vi "CAN发车速.vi"() -> ()   [LabVIEW 2020]
uses:
  Other/ZLG_CAN/Snap7/lib/Snap7.lvlib
  Other/ZLG_CAN/ZLG_CAN.lvlib
panel:
  in  "周期(ms)":u32=10 min=1 format="%d ms"
  in  "帧格式":enum16{"数据帧", "远程帧"}(ring)
  in  "帧类型":enum8{"标准帧", "扩展帧"}(ring)
  in  "ID":u32 format="0x%x"
  in  "波特率":u32(ring)=11 items=["5Kbps", "10Kbps", "20Kbps", "40Kbps", "50Kbps", "80Kbps", "100Kbps", "125Kbps", "200Kbps", "250Kbps", "400Kbps", "500Kbps", "666Kbps", "800Kbps", "1000Kbps"]
  in  "CAN 通道":u32(ring) items=["0", "1"]
  in  "索引":u32(ring) items=["0", "1", "2", "3", "4", "5", "6", "7", "8"]
  in  "设备类型":u32(ring)=3 items=["PCI5121"=1, "PCI9810"=2, "USBCAN1"=3, "USBCAN2"=4, "PCI9820"=5, "PCI5110"=7, "PC104CAN"=11, "CANETUDP"=12, "PCI9840B"=14, "PC104C2"=15, "PCI9820I"=16, "CANETTCP"=17, "PCIE9221"=24, "PCI5010U"=19, "USBCAN_E_U"=20, "USBCAN_2E_U"=21, "PCI5020U"=22, "PCIE9120I"=27, "PCIE9110I"=28, "PCIE9140I"=29]
  out "?":string
  out "Running":bool
  out "Status":string="No Error"
  in  "Word Length":i32(ring)=2 items=["Bit"=1, "Byte"=2, "Word"=4, "DWord"=6, "Real"=8, "Counter"=28, "Timer"=29]
  in  "Area":i32(ring)=132 items=["Inputs (EB)"=129, "Output (AB)"=130, "Bit Memory (M)"=131, "Data (DB)"=132, "Counters (Z)"=28, "Timers (T)"=29]
  in  "Amount":i32=1
  in  "Start":i32
  in  "DB Number":i32=1
  out "Data":u8[](array[numeric])
  in  "Stop":bool
  in  "Slot":i32=1
  in  "Rack":i32
  in  "Address IP":string="192.168.0.21"
  # "Data Read"
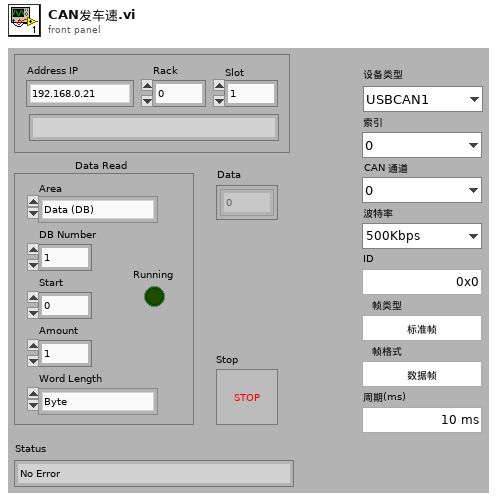
[diagram p1: front panel]
types:
  T1 = enum16{"big-endian, network order", "native, host order", "little-endian"}
  T2 = typedef "ZLG_CAN.lvlib/Start_CAN (Reply Payload)--cluster.ctl" = cluster{"Success":bool, "Start_CAN_error":errorcluster}
  T3 = cluster{u8, u8, "y":u8, "y":u8, "y":u8, "y":u8, "y":u8, "y":u8}
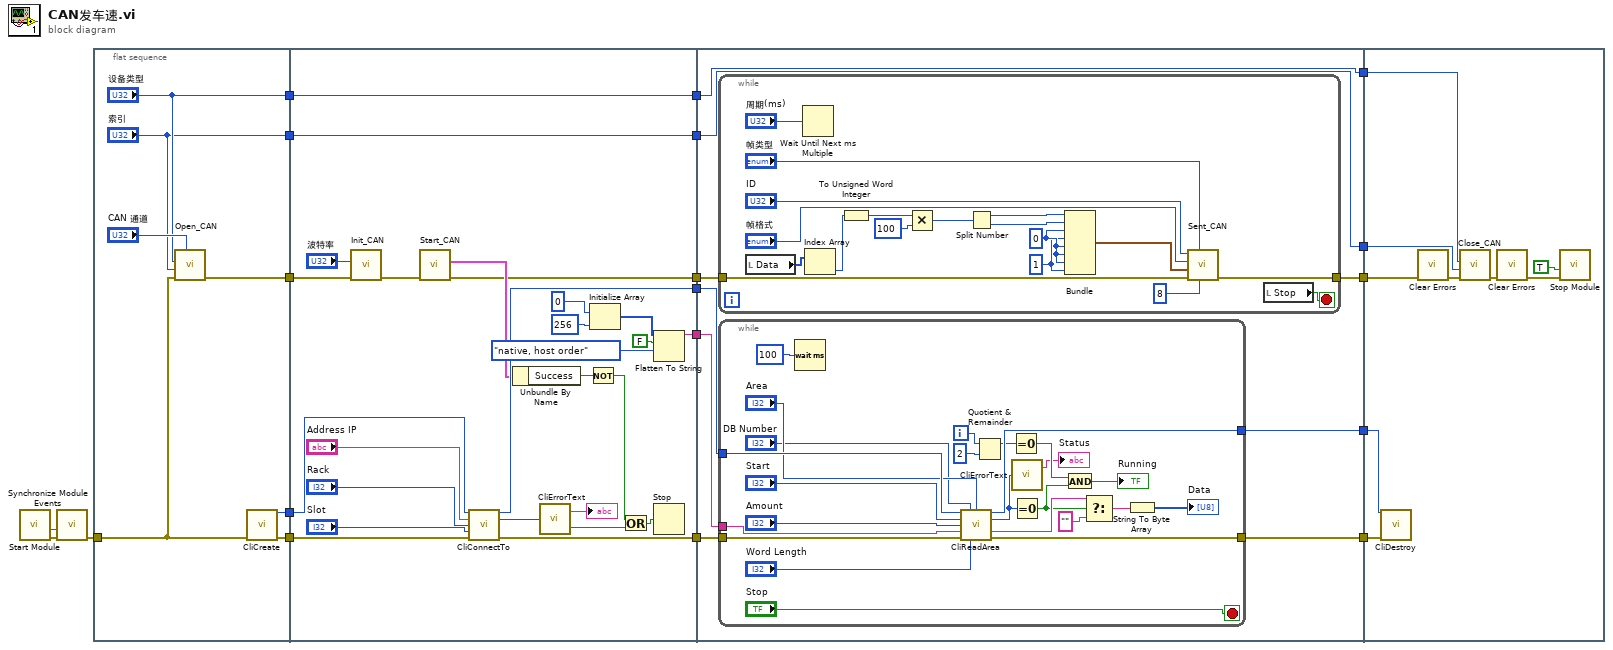
[diagram p0: block diagram]
diagram:
  n1 = call "Start Module.vi"() -> ("error out"=w12:errorcluster, "Wait for Event Sync?"=w11:bool)  [unwired: 8 in, 2 out]
  n2 = call "Synchronize Module Events.vi"("error in (no error)"=w12, "Wait for Event Sync?"=w11) -> ("error out"=w10:errorcluster)  [unwired: 9 in]
  n3 = flat-sequence {
    tunnel: [w26] -> w16
    tunnel: [w25] -> w15
    tunnel: w10 -> [w21]
    tunnel: ["索引"] -> w3
    tunnel: ["设备类型"] -> w2
    tunnel: [w22] -> w1
    tunnel: [w47] -> w19
    tunnel: [w40] -> w18
    tunnel: [w46] -> w17
    tunnel: w16 -> [w42]
    tunnel: w15 -> [w41]
    tunnel: [w36] -> w9
    tunnel: [w30] -> w7
    tunnel: [w31] -> w5
    tunnel: w3 -> [w31]
    tunnel: w2 -> [w30]
    tunnel: w1 -> [w29]
    tunnel: w19 -> [w61]
    tunnel: w18 -> [w60]
    tunnel: w17 -> [w59]
    tunnel: [w58] -> w14
    tunnel: [w57] -> w13
    tunnel: w9 -> [w56]
    tunnel: [w55] -> w8
    tunnel: w7 -> [w54]
    tunnel: [w54] -> w6
    tunnel: w5 -> [w53]
    tunnel: [w53] -> w4
    tunnel: w14 -> [w112]
    tunnel: w13 -> [w111]
    tunnel: w8 -> [w110]
    tunnel: w6 -> [w109]
    tunnel: w4 -> [w108]
    frame #0 {
      n4 = call "Open_CAN.vi"("CAN 通道"="CAN 通道", "error in (no error)"=w21, "索引"="索引", "设备类型"="设备类型") -> ("error out"=w22:errorcluster)  [unwired: 7 in]
      n5 = call "CliCreate.vi"("error in (no error)"=w21) -> ("ref out"=w26:u64, "error out"=w25:errorcluster)  [unwired: 13 in]
    }
    frame #1 {
      n6 = call "Init_CAN.vi"("error in (no error)"=w29, "波特率"="波特率") -> ("error out"=w32:errorcluster)  [unwired: 9 in]
      n7 = call "Start_CAN.vi"("error in (no error)"=w32) -> ("error out"=w36:errorcluster, "Reply Payload"=w37:T2)  [unwired: 8 in, 1 out]
      n8 = call "CliConnectTo.vi"("ref in"=w42, "Address"="Address IP", "Rack"="Rack", "Slot"="Slot", "error in (no error)"=w41) -> ("ref out"=w40:u64, "Result"=w38:i32, "error out"=w47:errorcluster)  [unwired: 8 in]
      n9 = Unbundle By Name(w37) -> ("Success"=w35:bool)
      n10 = call "CliErrorText.vi"("ErrNo"=w38) -> ("Error"=w34:bool, "ErrMessage"=→"?":string)
      n11 = Not(x=w35) -> (.not. x?=w27:bool)
      n12 = Initialize Array(u8 0, 256) -> (w50:u8[])
      n13 = Or(x=w27, y=w34) -> (x .or. y?=w33:bool)
      n14 = Flatten To String(anything=w50, prepend array or string size? (T)=FALSE, byte order (0:big-endian, network order)=T1."native, host order") -> (data string=w46:string)  [unwired: 1 in, 2 out]
      n15 = Stop(stop? (T)=w33) -> ()
    }
    frame #2 {
      n16 = while {
        tunnel: w56 -> [w79]
        tunnel: [w77] -> w55
        stop <- w78 stop-if-true
        w68 = u8 1 ("y")
        w69 = u8 0 ("y")
        n17 = local read "Data"() -> (w76:u8[])
        n18 = Wait Until Next ms Multiple(millisecond multiple="周期(ms)") -> ()  [unwired: 1 out]
        n19 = Index Array(array=w76) -> (element=w75:u8)  [unwired: 1 in]
        n20 = To Unsigned Word Integer(number=w75) -> (unsigned 16bit integer=w73:u16)
        n21 = Multiply(x=w73, y=u16 100) -> (x*y=w72:u16)
        n22 = Split Number(x=w72) -> (hi(x)=w71:u8, lo(x)=w70:u8)
        n23 = Bundle(w71, w70, "y"=w69, "y"=w68, "y"=w69, "y"=w69, "y"=w69, "y"=w68) -> (w67:T3)  [unwired: 1 in]
        n24 = call "Sent_CAN.vi"("帧长度"=u8 8, "帧类型"="帧类型", "error in (no error)"=w79, "帧数据"=w67, "帧格式"="帧格式", "ID"="ID") -> ("error out"=w77:errorcluster)  [unwired: 5 in]
        n25 = local read "Stop"() -> (w78:bool)
      }
      n26 = while {
        tunnel: w61 -> [w102]
        tunnel: w60 -> [w101]
        tunnel: w59 -> [w100]
        tunnel: [w94] -> w58
        tunnel: [w93] -> w57
        i -> [w91]
        stop <- "Stop" stop-if-true
        n27 = Wait (ms)(milliseconds to wait=u32 100 ("Loop Delay (ms)")) -> ()  [unwired: 1 out]
        n28 = call "CliReadArea.vi"("ref in"=w101, "DB Number"="DB Number", "Area"="Area", "Start"="Start", "Amount"="Amount", "data in"=w100, "error in (no error)"=w102, "Word Length"="Word Length") -> ("ref out"=w94:u64, "Result"=w92:i32, "data out"=w85:string, "error out"=w93:errorcluster)  [unwired: 4 in]
        n29 = Quotient & Remainder(x=w91, y=2) -> (x-y*floor(x/y)=w89:i32)  [unwired: 1 out]
        n30 = Equal To 0?(x=w89) -> (x = 0?=w88:bool)
        n31 = call "CliErrorText.vi"("ErrNo"=w92) -> ("ErrMessage"=→"Status":string)  [unwired: 1 out]
        n32 = Equal To 0?(x=w92) -> (x = 0?=w84:bool)
        n33 = And(x=w88, y=w84) -> (x .and. y?=→"Running":bool)
        n34 = Select(t=w85, s=w84, f="") -> (s? t:f=w82:string)
        n35 = String To Byte Array(string=w82) -> (unsigned byte array=→"Data":u8[])
      }
    }
    frame #3 {
      n36 = call "CliDestroy.vi"("ref in"=w112, "error in (no error)"=w111) -> ()  [unwired: 13 in, 1 out]
      n37 = call <vilib>:"Clear Errors.vi"("error in (no error)"=w110) -> ("error out"=w104:errorcluster)  [unwired: 5 in, 1 out]
      n38 = call "Close_CAN.vi"("error in (no error)"=w104, "索引"=w108, "设备类型"=w109) -> ("error out"=w107:errorcluster)  [unwired: 8 in]
      n39 = call <vilib>:"Clear Errors.vi"("error in (no error)"=w107) -> ("error out"=w105:errorcluster)  [unwired: 5 in, 1 out]
      n40 = call "Stop Module.vi"("error in (no error)"=w105, "Wait for Module to Stop? (F)"=TRUE) -> ()  [unwired: 9 in, 1 out]
    }
  }
